vi "Add New UI Reference.vi"(8 "error in (no error)":errorcluster, 9 "Name":string, 10 "VI Refnum":refnum<vi>, 11 "UI Reference Wrapper in":refnum<class "UI Reference Wrapper.lvclass">) -> (0 "error out":errorcluster, 3 "UI Reference Wrapper out":refnum<class "UI Reference Wrapper.lvclass">)   [LabVIEW 2014, in "UI Reference Wrapper.lvclass"]
uses:
  UI Reference Wrapper.lvclass
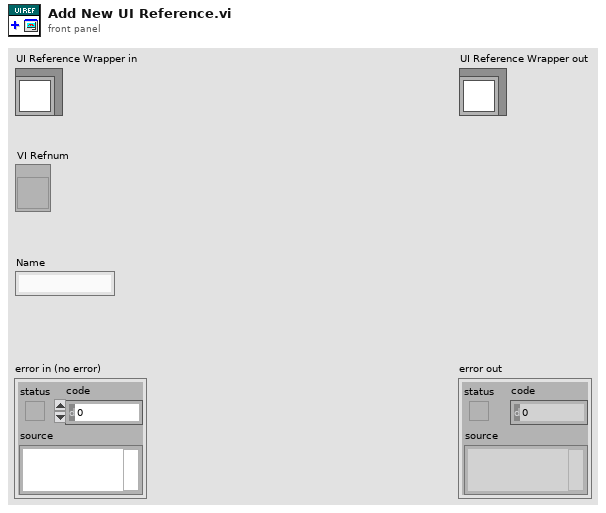
[diagram p1: front panel]
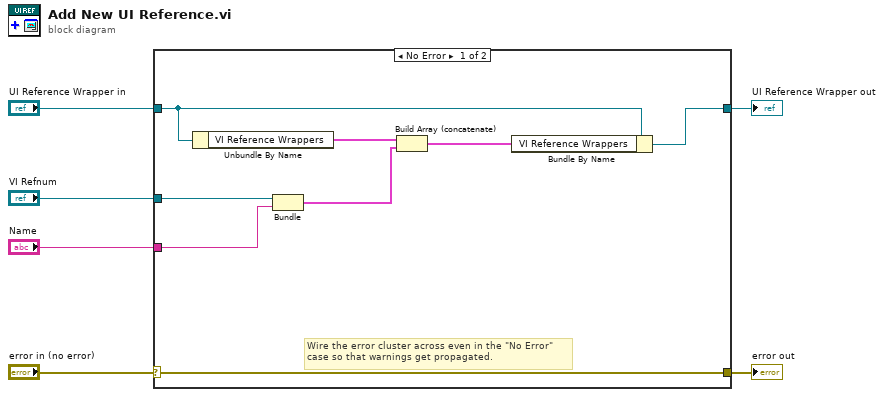
[diagram p0: block diagram]
diagram:
  n1 = case shown="No Error" "error in (no error)" {
    selector: "error in (no error)" -> [w14 w16]
    tunnel: [w14 w16] -> w5
    tunnel: [w12 w15] -> w3
    tunnel: "UI Reference Wrapper in" -> [w13 w15]
    tunnel: "VI Refnum" -> [w9 _]
    tunnel: "Name" -> [w8 _]
    frame No Error {
      # "Wire the error cluster across even in the \"No Error\"\ncase so that warnings get propagated."
      n2 = Unbundle By Name(w13) -> ("VI Reference Wrappers"=w11:cluster{"VI Refnum":refnum<vi>, "Name":string}[])
      n3 = Bundle("VI Refnum"=w9, "Name"=w8) -> (w7:cluster{"VI Refnum":refnum<vi>, "Name":string})  [unwired: 1 in]
      n4 = Build Array (concatenate)(w11, w7) -> (w10:cluster{"VI Refnum":refnum<vi>, "Name":string}[])
      n5 = Bundle By Name(cluster=w13, "VI Reference Wrappers"=w10) -> (w12:refnum<class "UI Reference Wrapper.lvclass">)
    }
    frame Error {
    }
  }
  "error out" <- w5
  "UI Reference Wrapper out" <- w3
